vi "Run-TimePosition.Centered.vi"(8 "error in (no error)":errorcluster, 9 "Size":cluster{"Height":i16, "Width":i16}, 10 "Monitor":i16, 11 "WindowFrame in":refnum<class "WindowFrame.lvclass">) -> (0 "error out":errorcluster, 3 "WindowFrame out":refnum<class "WindowFrame.lvclass">)   [LabVIEW 2021, in "WindowFrame.lvlib" / "WindowFrame.lvclass"]
uses:
  WindowFrame.lvclass
  FrontPanel.Run-TimePosition.Centered.ctl
  Action.ctl
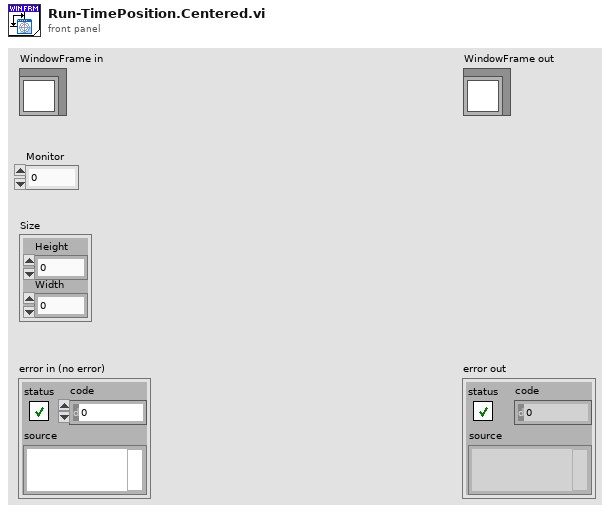
[diagram p1: front panel]
types:
  T1 = typedef "WindowFrame.lvlib/WindowFrame.lvclass/FrontPanel.Run-TimePosition.Centered.ctl" = cluster{"Monitor":i16, "Size":cluster{"Height":i16, "Width":i16}}
  T2 = typedef "WindowFrame.lvlib/WindowFrame.lvclass/Action.ctl" = enum16{"Set Allow Runtime PopUp", "Set Behavior", "Set Closable", "Set Custom Title", "Set Highlight Return Button", "Set Is Frontmost", "Set Minimizable", "Set Minimum Size", "Set Monitor", "Set Resizable", "Set Panel Bounds", "Set Run VI Transparently", "Set Show Menu Bar", "Set State", "Set Title", "Set Title Bar Colors", "Set Title Bar Visible", "Set Transparancy", "Set Window Bounds", "Get Allow Runtime PopUp", "Get Behavior", "Get Closable", "Get Custom Title", "Get Highlight Return Button", "Get Is Frontmost", "Get Minimizable", "Get Minimum Size", "Get Monitor", "Get Panel Bounds", "Get Resizable", "Get Run VI Transparently", "Get Show Menu Bar", "Get State", "Get Title", "Get Title Bar Colors", "Get Title Bar Visible", "Get Transparancy", "Get Window Bounds", "--", "Center", "Close", "Open", "Run-Time Position:Centered", "Run-Time Position:Custom", "Run-Time Position:Get Position", "Run-Time Position:Maximized", "Run-Time Position:Minimized", "Run-Time Position:Unchanged", "---", "Insert VI", "Remove VI", "Insert VI Index", "Remove VI Index", "Exit"}
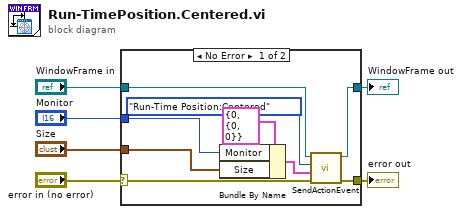
[diagram p0: block diagram]
diagram:
  n1 = case shown="No Error" "error in (no error)" {
    selector: "error in (no error)" -> [w13 w17]
    tunnel: [w12 w17] -> w5
    tunnel: [w15 w16] -> w3
    tunnel: "WindowFrame in" -> [w14 w16]
    tunnel: "Monitor" -> [w11 _]
    tunnel: "Size" -> [w7 _]
    frame No Error {
      n2 = Bundle By Name(cluster=T1 {"Monitor"=0, "Size"={"Height"=0, "Width"=0}}, "Monitor"=w11, "Size"=w7) -> (w9:T1)
      n3 = call "SendActionEvent.vi"("error in (no error)"=w13, "Variant"=w9, "Action"=Action."Run-Time Position:Centered", "WindowFrame in"=w14) -> ("error out"=w12:errorcluster, "WindowFrame out"=w15:refnum<class "WindowFrame.lvclass">)  [unwired: 6 in]
    }
    frame Error {
    }
  }
  "error out" <- w5
  "WindowFrame out" <- w3
